vi "Update Configuration Command.vi"(8 "error in":errorcluster, 10 "Config JSON":string, 11 "CIFCorePlugin in":refnum<class "CIFCorePlugin.lvclass">) -> (0 "error out":errorcluster, 3 "CIFCorePlugin out":refnum<class "CIFCorePlugin.lvclass">)   [LabVIEW 2021, in "CIFCorePlugin.lvclass"]
uses:
  CIFCorePlugin.lvclass
  Typedef/gRPC to Main Commands.ctl
  <vilib>/addons/_JKI.lib/Serialization/JSON/JKI JSON Serialization.lvlib
  7a6034d4-97b5-44d3-b8f0-d6743db7723f.vi
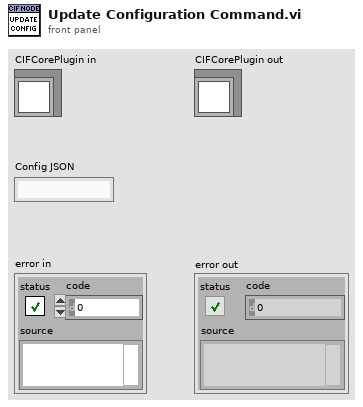
[diagram p1: front panel]
types:
  T1 = typedef "CIFCorePlugin.lvclass/gRPC to Main Commands.ctl" = enum8{"Start", "Pause", "Stop", "RefreshStats", "UpdateConfig", "Update Clock Map", "Connect Channel", "Force Channel", "Add Publisher Instance", "Remove Publisher Instance"}
  T2 = typedef "CIFCorePlugin.lvclass/gRPC to Main DVR.ctl" = refnum<data-value>
  T3 = typedef "CIFCoreCommon.lvlib/gRPC to Main Data.ctl" = cluster{"Config Data":variant, "Connection":T4, "Force":T5, "Clock Conversion":T6, "Publisher Instance":T8}
  T4 = typedef "CIFCoreCommon.lvlib/Channel Connection Data.ctl" = cluster{"Publisher Name":string, "Subscriber Name":string, "Connection Data":u8[]}
  T5 = typedef "CIFCoreCommon.lvlib/Channel Force Data.ctl" = cluster{"Channel Name":string, "Force Data":u8[], "Force Active":bool}
  T6 = typedef "Time_CIF_U.lvlib/Clock Conversion Map.ctl" = map{u8, cluster{"Last Reset":i64, "Offset Pair":T7, "Slope":dbl, "1/Slope":dbl}}
  T7 = typedef "Time_CIF_U.lvlib/Timestamp Pair.ctl" = cluster{"System Time":i64, "External Time":i64}
  T8 = typedef "CIFCoreCommon.lvlib/FIFO Publisher.ctl" = cluster{"Publisher Name":string, "New FIFO Instance Config":T9}
  T9 = typedef "ChannelCommon.lvlib/New FIFO Instance Configuration.ctl" = cluster{"Primary":bool, "Backpressure":bool, "Message/FIFO Override":u32}
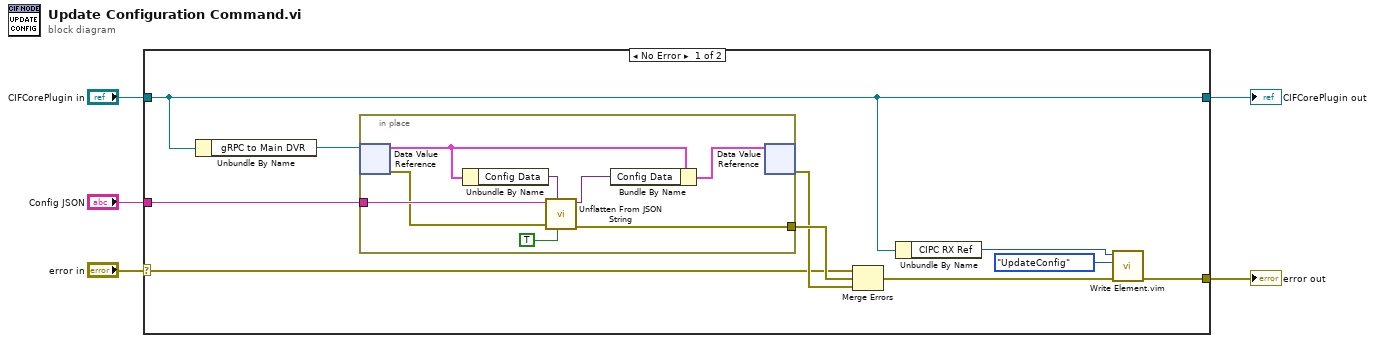
[diagram p0: block diagram]
diagram:
  n1 = case shown="No Error" "error in" {
    selector: "error in" -> [w6 w25]
    tunnel: [w14 w25] -> w4
    tunnel: "CIFCorePlugin in" -> [w12 w24]
    tunnel: [w12 w24] -> w2
    tunnel: "Config JSON" -> [w10 _]
    frame No Error {
      n2 = Unbundle By Name(w12) -> ("gRPC to Main DVR"=w11:T2)
      n3 = in-place {
        in-place-border: w10 -> [w19]
        in-place-border: [w18] -> w9
        n4 = in-place-dvr #1(w11) -> (w20:T3, w16:errorcluster)
        n5 = Unbundle By Name(w20) -> ("Config Data"=w23:variant)
        n6 = call <vilib>:"Unflatten From JSON String.vi"("Nulls as Defaults (F)"=TRUE, "Type and Defaults"=w23, "error in (no error)"=w16, "JSON String"=w19) -> ("error out"=w18:errorcluster, "Variant"=w21:variant)  [unwired: 6 in]
        n7 = Bundle By Name(cluster=w20, "Config Data"=w21) -> (w17:T3)
        n8 = in-place-dvr #1(w17) -> (w8:errorcluster)  [unwired: 1 out]
      }
      n9 = Merge Errors(w6, w9, w8) -> (w7:errorcluster)
      n10 = Unbundle By Name(w12) -> ("CIPC RX Ref"=w13:u64)
      n11 = call "Write Element.vim"("error in (no error)"=w7, "Data in"=gRPC_to_Main_Commands."UpdateConfig" ("OOB Main Commands"), "CIPC Reference in"=w13) -> ("error out"=w14:errorcluster)  [unwired: 5 in, 3 out]
    }
    frame Error {
    }
  }
  "error out" <- w4
  "CIFCorePlugin out" <- w2
